vi "Autosort Parameter Set selected.vi"(9 "NewVal":i8, 10 "Data OUT":T1={"Impulse Positions"=[], "Old Impulse positions for Undo"=[], "No. Imp"=0, "Parameter Time Series"=[], "Parameter Impuls Series"=[], "Experiment Parameters"={"Freq"=0.0, "Vel"=0, "Acc"=0, "Stimulus"=""}, "Autosort File"=refnum, "Data File"={"Data Channels"=[], "Sample Rate"=0, "Channel List"=[]}, "Experiment data path"=path "", "Image data path"=path "", "LVS data path"=path "", "Raw copy path"=path "", "filename"="", "desaccading parameters"={"Tolerance"=0, "Acc Range"=0.0, "Sample Rate"=0, "Impulse Plane 2"=enum."Other", "Impulse dir"=FALSE}, "Experiment Parameters 2"={"Subject"="", "Strain"="", "Rotation plane"="", "Experimenter"="", "Trial"=0.0, "Time"=0.0}, "Excel"={"Excel._Application"=refnum, "Use Excel"=FALSE, "Worksheet SINE"=refnum, "Row SINE"=0, "Worksheet TRANS"=refnum, "Row TRANS"=0}, "Session Config File"=refnum, "Autosort Parameter Set"=0, "EMA Version"="", "desacc "={"Threshold 1 [Acc]"=0.0, "Threshold 2 [% of TH1]"=0, "tolerance"=0, "Search WD "=0.0, " always use TH2"=FALSE, "Range"=0.0, "Max time"=0.0, "Min time"=0.0, "Velocity Threshold"=0}, "Cycle Nr for Saccades"={"POS"=0, "NEG"=0}, "Undo Counter"=0, "History Length"=0, "Redo Counter"=0, "Histpry Position"=0, "Raw Data File"={"Data Channels"=[], "Sample Rate"=0, "Channel List"=[]}, "calibration name"="No file selected"} {"Parameter Time Series"."time offset" format="%.3f"; "Parameter Time Series"."Gain" format="%.1f"; "Parameter Time Series"."Offset" format="%.1f"; "Parameter Time Series"."List 1" items=["Motor-Pos", "Motor-Vel", "Lx Position-in-Head", "Ly Position-in-Head", "Lz Position-in-Head", "Lx Velocity-in-Head", "Ly Velocity-in-Head", "Lz Velocity-in-Head", "Ll Velocity-in-Head", "Lr Velocity-in-Head", "Lx Accel-in-Head", "Ly Accel-in-Head", "Lz Accel-in-Head", "Rx Position-in-Head", "Ry Position-in-Head", "Rz Position-in-Head", "Rx Velocity-in-Head", "Ry Velocity-in-Head", "Rz Velocity-in-Head", "Rl Velocity-in-Head", "Rr Velocity-in-Head", "Rx Accel-in-Head", "Ry Accel-in-Head", "Rz Accel-in-Head", "Global Trigger", "", "", ""]; "Parameter Impuls Series"."Gain" format="%.1f"; "Parameter Impuls Series"."Offset" format="%.1f"}, 11 "Ring in":refnum<vi>) -> (3 "State stack IN":T4[](array[typedef]))   [LabVIEW 2016]
uses:
  private/Impulse Analyser state.ctl
  type-defs/TD_Statemachine-Data.ctl
  type-defs/TD_Time Series.ctl
  type-defs/TD_Impulse Parameter.ctl
  plugins/Mars 3D/Mars3D_autosort.vi
  core.lvlib
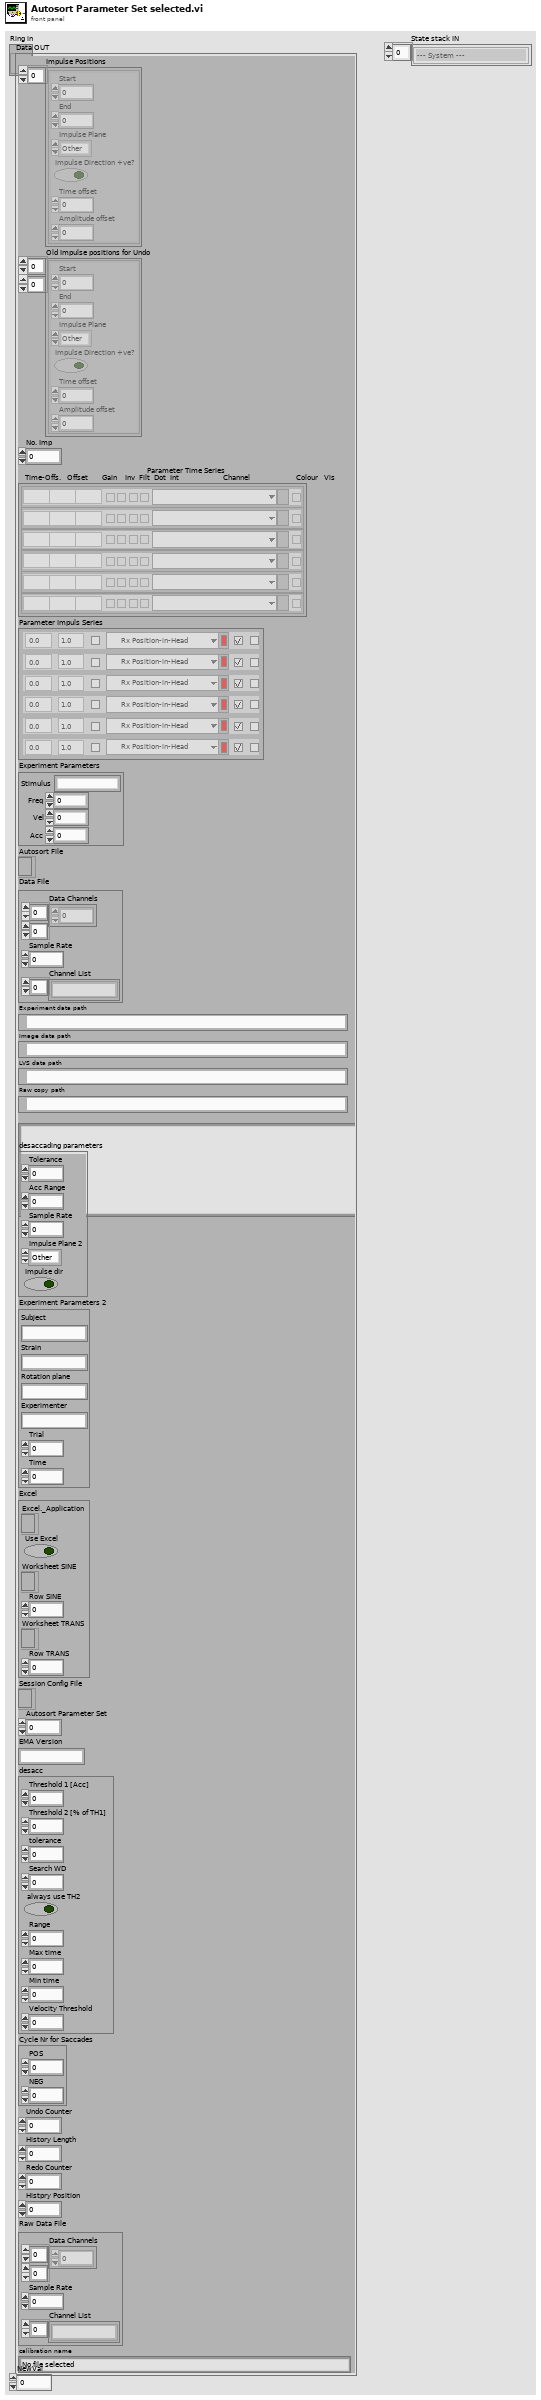
[diagram p1: front panel]
types:
  T1 = typedef "core.lvlib/TD_Statemachine-Data.ctl" = cluster{"Impulse Positions":cluster{"Start":i32, "End":i32, "Impulse Plane":enum16{"Other", "Yaw", "Pitch", "Roll", "LARP", "RALP"}, "Impulse Direction +ve?":bool, "Time offset":i32, "Amplitude offset":dbl}[], "Old Impulse positions for Undo":cluster{"Start":i32, "End":i32, "Impulse Plane":enum16{"Other", "Yaw", "Pitch", "Roll", "LARP", "RALP"}, "Impulse Direction +ve?":bool, "Time offset":i32, "Amplitude offset":dbl}[][], "No. Imp":i32, "Parameter Time Series":T2, "Parameter Impuls Series":T3, "Experiment Parameters":cluster{"Freq":dbl, "Vel":i32, "Acc":i32, "Stimulus":string}, "Autosort File":refnum<file>, "Data File":cluster{"Data Channels":dbl[][], "Sample Rate":i32, "Channel List":string[]}, "Experiment data path":path, "Image data path":path, "LVS data path":path, "Raw copy path":path, "filename":string, "desaccading parameters":cluster{"Tolerance":i32, "Acc Range":dbl, "Sample Rate":i32, "Impulse Plane 2":enum16{"Other", "Yaw", "Pitch", "Roll", "LARP", "RALP"}, "Impulse dir":bool}, "Experiment Parameters 2":cluster{"Subject":string, "Strain":string, "Rotation plane":string, "Experimenter":string, "Trial":dbl, "Time":dbl}, "Excel":cluster{"Excel._Application":refnum<k7>, "Use Excel":bool, "Worksheet SINE":refnum<k7>, "Row SINE":i32, "Worksheet TRANS":refnum<k7>, "Row TRANS":i32}, "Session Config File":refnum<file>, "Autosort Parameter Set":i32, "EMA Version":string, "desacc ":cluster{"Threshold 1 [Acc]":dbl, "Threshold 2 [% of TH1]":i32, "tolerance":i32, "Search WD ":dbl, " always use TH2":bool, "Range":dbl, "Max time":dbl, "Min time":dbl, "Velocity Threshold":i32}, "Cycle Nr for Saccades":cluster{"POS":i32, "NEG":i32}, "Undo Counter":i32, "History Length":i32, "Redo Counter":i32, "Histpry Position":i32, "Raw Data File":cluster{"Data Channels":dbl[][], "Sample Rate":i32, "Channel List":string[]}, "calibration name":string}
  T2 = typedef "core.lvlib/TD_Time Series.ctl" = cluster{"time offset":dbl, "Offset":dbl, "Gain":dbl, "inverse":bool, "filter data":bool, "dots":bool, "interpolate":bool, "List 1":u16, "Color Box":u32, "Boolean":bool}[]
  T3 = typedef "core.lvlib/TD_Impulse Parameter.ctl" = cluster{"Color":u32, "Visible":bool, "Channel":u16, "Invert":bool, "Desaccade":bool, "Offset":dbl, "Gain":dbl}[]
  T4 = typedef "Impulse Analyser state.ctl" = enum16{"--- System ---", "Panel Monitoring", "Check Save Status", "Initialize", "Initialise GUI", "Quit", "--- Import ---", "Desaccade Time Data", "Desaccade Time Data Background", "Paint Delete", "Load Batch Log File", "Make Batch List", "Update Batch List", "Delete Batch List", "Delete Temporary LVS", "Save Temporary LVS", "Check for Batch LVS", "Process 3D Chinchilla", "Find default parameter", "Mars3D old", "Chair", "EyeSeeCam", "Open last session", "Save RAW", "Auto Impulse Parameter", "Save Image", "Wireless", "Process Coils Data", "Process JHOC Data", "Process Animal Data", "Australian Data", "ASCII", "Mars 3D", "Mars 3D Training", "Position Mean Plugin", "plot generator plugin", "Human VOG system", "Optotrak", "spline", "COR", "galvanic", "Generate New Time Plot", "Make off and gains permanent", "Generate New Impulse Plot", "Snap Impulse Cursor", "Extract Saccades", "Impulse Analyser", "NTA", "Acceleration", "Saccade Velocity", "Horizontal Align", "Vertical Align", "Delete Impulse", "Cut Before", "Cut After", "Filter Data", "Undo Last", "Redo", "Mean and STD", "Group Analyser", "Generate Report", "Phase Plots", "Gain and Phase", "Example Plugin", "Time Constant Plugin", "Export Data", "Export Time Series Data", "Append Data", "Save Data", "Load Data", "Cut in Range", "Keep in range", "Stop"}
  T5 = cluster{"Autosize Parameter Set 2":cluster{"Trigger Ch":i32, "Min Vel":dbl, "MaxVel":dbl, "Width":i32, "Pre Impuls":i32, "Post Impuls":i32, "Pitch":dbl, "Name":string, "Other Trigger":bool, "Cross Corr":bool, "Default":cluster{"Freq":dbl, "Vel":dbl, "Acc":dbl, "Stimulus":string}}[]}[]
  T6 = cluster{"Autosize Parameter Set 2":cluster{"Trigger Ch":i32, "Min Vel":dbl, "MaxVel":dbl, "Width":i32, "Pre Impuls":i32, "Post Impuls":i32, "Pitch":dbl, "Name":string, "Other Trigger":bool, "Cross Corr":bool, "Default":cluster{"Freq":dbl, "Vel":dbl, "Acc":dbl, "Stimulus":string}}[]}
  T7 = cluster{"Trigger Ch":i32, "Min Vel":dbl, "MaxVel":dbl, "Width":i32, "Pre Impuls":i32, "Post Impuls":i32, "Pitch":dbl, "Name":string, "Other Trigger":bool, "Cross Corr":bool, "Default":cluster{"Freq":dbl, "Vel":dbl, "Acc":dbl, "Stimulus":string}}[]
  T8 = cluster{"Freq":dbl, "Vel":i32, "Acc":i32, "Stimulus":string}
  T9 = cluster{"Freq":dbl, "Vel":dbl, "Acc":dbl, "Stimulus":string}
  T10 = cluster{"Freq":bool, "Vel":bool, "Acc":bool, "Stimulus":bool}
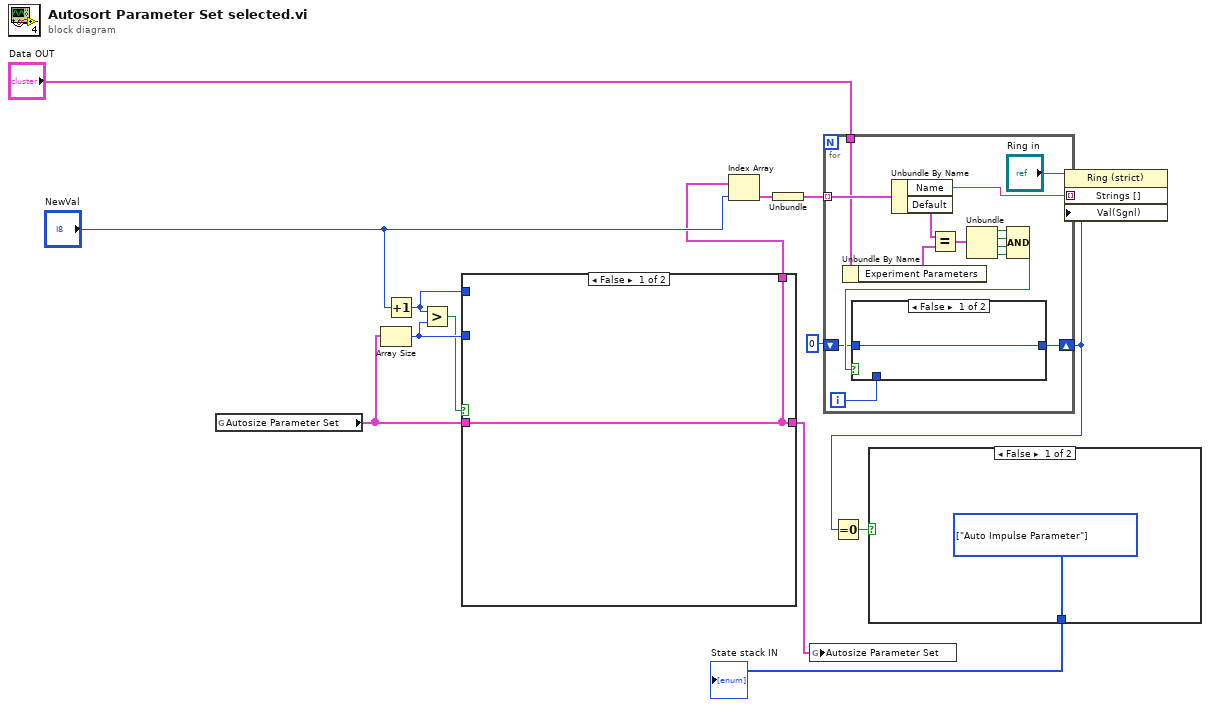
[diagram p0: block diagram]
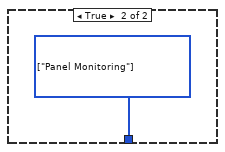
[diagram p2: hidden frame]
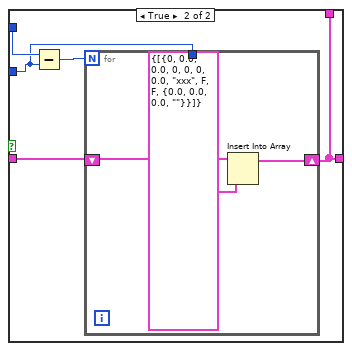
[diagram p3: hidden frame]
diagram:
  n1 = global read "Mars3D_autosort.vi" "Autosize Parameter Set"() -> (w4:T5)
  n2 = Array Size(array=w4) -> (size(s)=w6:i32)
  n3 = Increment(x="NewVal") -> (x+1=w8:i8)
  n4 = Greater?(x=w8, y=w6) -> (0:w3:bool)
  n5 = case shown="False" w3 {
    tunnel: w6 -> [_ w20]
    tunnel: w4 -> [w17 w22]
    tunnel: [w17 w19] -> w5
    tunnel: w8 -> [_ w21]
    tunnel: [w17 w19] -> w7
    frame False {
    }
    frame True {
      n6 = Subtract(x=w21, y=w20) -> (x-y=w18:i32)
      n7 = for {
        N: w18 -> [_]
        tunnel: w20 -> [_]
        shift-right: [w25] -> w19
        shift-left: w22 -> [w24]
        n8 = Insert Into Array(array=w24, new element=T6 {"Autosize Parameter Set 2"=[{"Trigger Ch"=0, "Min Vel"=0.0, "MaxVel"=0.0, "Width"=0, "Pre Impuls"=0, "Post Impuls"=0, "Pitch"=0.0, "Name"="xxx", "Other Trigger"=FALSE, "Cross Corr"=FALSE, "Default"={"Freq"=0.0, "Vel"=0.0, "Acc"=0.0, "Stimulus"=""}}]} ("new element/subarray")) -> (w25:T5)  [unwired: 1 in]
      }
    }
  }
  n9 = Index Array(array=w5, index="NewVal") -> (element=w10:T6)
  n10 = Unbundle(w10) -> ("Autosize Parameter Set 2"=w11:T7)
  n11 = global write "Mars3D_autosort.vi" "Autosize Parameter Set"(w7) -> ()
  n12 = for {
    tunnel: [w39] -> w2 mode=indexing
    tunnel: w11 -> [w38] mode=indexing
    tunnel: "Data OUT" -> [w36]
    shift-right: [w28] -> w14
    shift-left: 0 -> [w27]
    i -> [w26]
    n13 = Unbundle By Name(w36) -> ("Experiment Parameters"=w35:T8)
    n14 = Unbundle By Name(w38) -> ("Name"=w39:string, "Default"=w37:T9)
    n15 = Equal?(x=w37, y=w35) -> (x = y?=w34:T10)
    n16 = Unbundle(w34) -> ("Freq"=w33:bool, "Vel"=w32:bool, "Acc"=w31:bool, "Stimulus"=w30:bool)
    n17 = Compound Arithmetic op=AND(w33, w32, w31, w30) -> (w29:bool)
    n18 = case shown="False" w29 {
      tunnel: [w40 w41] -> w28
      tunnel: w27 -> [w40 _]
      tunnel: w26 -> [_ w41]
      frame False {
      }
      frame True {
      }
    }
  }
  n19 = Equal To 0?(x=w14) -> (x = 0?=w15:bool)
  n20 = case shown="False" w15 {
    tunnel: [w42 w43] -> w16
    frame False {
      w42 = T4[] [enum."Auto Impulse Parameter"] items=["--- System ---", "Panel Monitoring", "Check Save Status", "Initialize", "Initialise GUI", "Quit", "--- Import ---", "Desaccade Time Data", "Desaccade Time Data Background", "Paint Delete", "Load Batch Log File", "Make Batch List", "Update Batch List", "Delete Batch List", "Delete Temporary LVS", "Save Temporary LVS", "Check for Batch LVS", "Process 3D Chinchilla", "Find default parameter", "Mars3D old", "Chair", "EyeSeeCam", "Open last session", "Save RAW", "Auto Impulse Parameter", "Save Image", "Wireless", "Process Coils Data", "Process JHOC Data", "Process Animal Data", "Australian Data", "ASCII", "Mars 3D", "Mars 3D Training", "Position Mean Plugin", "plot generator plugin", "Human VOG system", "Optotrak", "spline", "COR", "galvanic", "Generate New Time Plot", "Make off and gains permanent", "Generate New Impulse Plot", "Snap Impulse Cursor", "Extract Saccades", "Impulse Analyser", "NTA", "Acceleration", "Saccade Velocity", "Horizontal Align", "Vertical Align", "Delete Impulse", "Cut Before", "Cut After", "Filter Data", "Undo Last", "Redo", "Mean and STD", "Group Analyser", "Generate Report", "Phase Plots", "Gain and Phase", "Example Plugin", "Time Constant Plugin", "Export Data", "Export Time Series Data", "Append Data", "Save Data", "Load Data", "Cut in Range", "Keep in range", "Stop"] ("State stack IN")
    }
    frame True {
      w43 = T4[] [enum."Panel Monitoring"] items=["--- System ---", "Panel Monitoring", "Check Save Status", "Initialize", "Initialise GUI", "Quit", "--- Import ---", "Desaccade Time Data", "Desaccade Time Data Background", "Paint Delete", "Load Batch Log File", "Make Batch List", "Update Batch List", "Delete Batch List", "Delete Temporary LVS", "Save Temporary LVS", "Check for Batch LVS", "Process 3D Chinchilla", "Find default parameter", "Mars3D old", "Chair", "EyeSeeCam", "Open last session", "Save RAW", "Auto Impulse Parameter", "Save Image", "Wireless", "Process Coils Data", "Process JHOC Data", "Process Animal Data", "Australian Data", "ASCII", "Mars 3D", "Mars 3D Training", "Position Mean Plugin", "plot generator plugin", "Human VOG system", "Optotrak", "spline", "COR", "galvanic", "Generate New Time Plot", "Make off and gains permanent", "Generate New Impulse Plot", "Snap Impulse Cursor", "Extract Saccades", "Impulse Analyser", "NTA", "Acceleration", "Saccade Velocity", "Horizontal Align", "Vertical Align", "Delete Impulse", "Cut Before", "Cut After", "Filter Data", "Undo Last", "Redo", "Mean and STD", "Group Analyser", "Generate Report", "Phase Plots", "Gain and Phase", "Example Plugin", "Time Constant Plugin", "Export Data", "Export Time Series Data", "Append Data", "Save Data", "Load Data", "Cut in Range", "Keep in range", "Stop"] ("State stack IN")
    }
  }
  "State stack IN" <- w16
  n21 = property on="Property Node" class="Ring (strict)"(reference="Ring in", "Strings []"=w2, "Val(Sgnl)"=w14) -> ()  [unwired: 1 in, 2 out]
